vi "KG set dry mode.vi"(8 "Fehler (Eingang, kein Fehler)":errorcluster, 10 "drywet":u32, 11 "VISA-Ressourcenname":refnum<visa-resource-name>) -> (0 "Fehler (Ausgang)":errorcluster, 2 "Komando gesendet":string, 3 "VISA-Ressourcenname (Ausgang)":refnum<visa-resource-name>)   [LabVIEW 2020, in "Linearisierung v2.lvlib" / "Gasteiler.lvlib" / "HovaCAL_Interface.lvlib" / "KGN.lvlib" / "set.lvlib"]
uses:
  set.lvlib
  KGN.lvlib
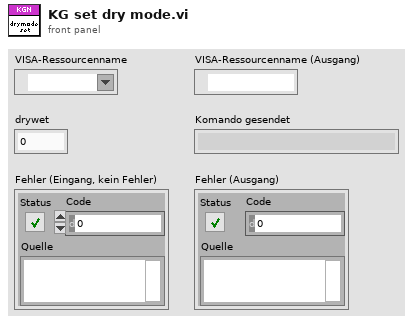
[diagram p1: front panel]
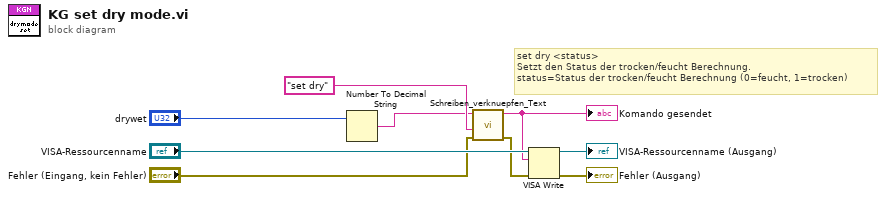
[diagram p0: block diagram]
diagram:
  # "set dry <status>\nSetzt den Status der trocken/feucht Berechnung.\nstatus=Status der trocken/feucht Berechnung (0=feucht, 1=trocken)"
  n1 = Number To Decimal String(number="drywet") -> (decimal integer string=w1:string)  [unwired: 1 in]
  n2 = call "Schreiben_verknuepfen_Text.vi"("error in (no error)"="Fehler (Eingang, kein Fehler)", "Order"="set dry" ("Schreibpuffer"), "parameter"=w1) -> ("error out"=w4:errorcluster, "Verknüpfter String"=w3:string)  [unwired: 7 in]
  "Komando gesendet" <- w3
  n3 = VISA Write(VISA resource name="VISA-Ressourcenname", write buffer=w3, error in (no error)=w4) -> (VISA resource name out=→"VISA-Ressourcenname (Ausgang)":refnum<visa-resource-name>, error out=→"Fehler (Ausgang)":errorcluster)  [unwired: 1 out]
